vi "Simulate_Model_(1 step).vi"(8 "error in (no error)":errorcluster, 11 "Model_Predictor in":refnum<class "Model_Predictor.lvclass">) -> (0 "error out":errorcluster, 3 "Model_Predictor out":refnum<class "Model_Predictor.lvclass">)   [LabVIEW 2021, in "MBPOnOff_Controller.lvlib" / "Model_Predictor.lvclass"]
uses:
  Model_Predictor.lvclass
  Model_Predictor.lvclass/Model_Predictor.ctl
  Get Current_Acting_control.vi
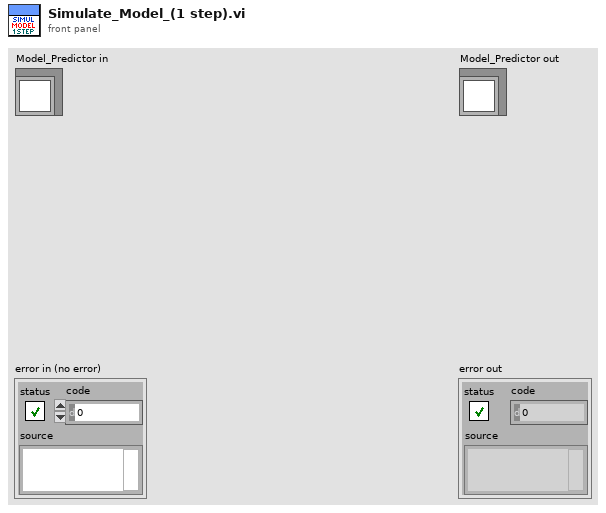
[diagram p1: front panel]
types:
  T1 = typedef "MBPOnOff_Controller.lvlib/Model_Predictor.lvclass/state_variables.ctl" = cluster{"So":dbl, "kLa":dbl}
  T2 = typedef "MBPOnOff_Controller.lvlib/Model_Predictor.lvclass/Model_v1_parameters.ctl" = cluster{"Sosat":dbl, "OUR":dbl, "R_OUR":dbl, "T_kLa":dbl, "R_T_kLa":dbl, "T0":dbl, "ku":dbl, "dt":dbl, "PWM total period":dbl, "PWM ON period":dbl, "OUR calc period":dbl, "OUR calc threshold":dbl}
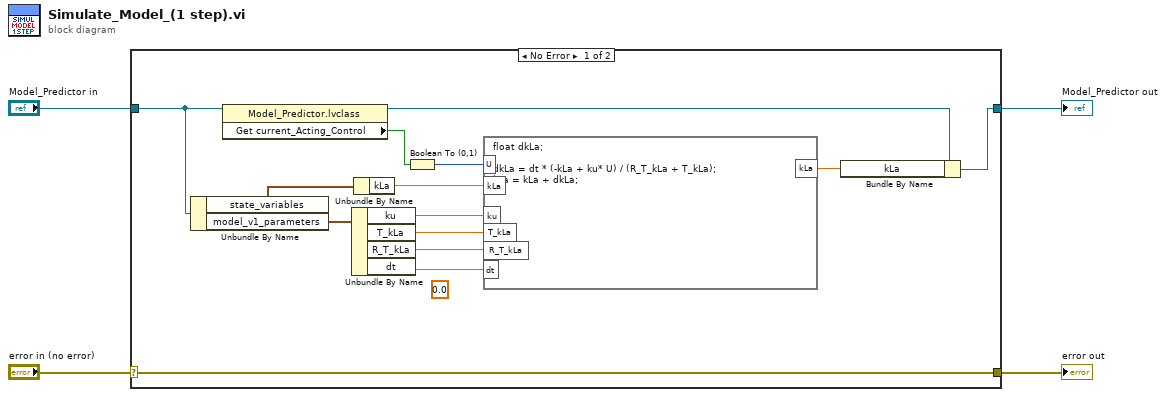
[diagram p0: block diagram]
diagram:
  n1 = case shown="No Error" "error in (no error)" {
    selector: "error in (no error)" -> [w18 w20]
    tunnel: [w18 w20] -> w3
    tunnel: [w16 w19] -> w1
    tunnel: "Model_Predictor in" -> [w17 w19]
    frame No Error {
      (unwired) 0.0 ("dt")
      n2 = Unbundle By Name(w17) -> ("state_variables"=w11:T1, "model_v1_parameters"=w14:T2)
      n3 = property class="Model_Predictor.lvclass"(reference=w17) -> (reference out=w15:refnum<class "Model_Predictor.lvclass">, "Get current_Acting_Control"=w13:bool)  [unwired: 1 in, 1 out]
      n4 = Unbundle By Name(w14) -> ("ku"=w7:dbl, "T_kLa"=w8:dbl, "R_T_kLa"=w9:dbl, "dt"=w5:dbl)
      n5 = Unbundle By Name(w11) -> ("kLa"=w10:dbl)
      n6 = Boolean To (0,1)(Boolean=w13) -> (0, 1=w12:i16)
      n7 = formula code="float dkLa;\n\ndkLa = dt * (-kLa + ku* U) / (R_T_kLa + T_kLa);\nkLa = kLa + dkLa;"("U"=w12, "ku"=w7, "kLa"=w10, "T_kLa"=w8, "R_T_kLa"=w9, "dt"=w5) -> ("kLa"=w6:dbl)
      n8 = Bundle By Name(cluster=w15, "kLa"=w6) -> (w16:refnum<class "Model_Predictor.lvclass">)
    }
    frame Error {
    }
  }
  "error out" <- w3
  "Model_Predictor out" <- w1
